vi "Test All Drivers.vi"() -> ()   [LabVIEW 2019, in "instrument.Cryostation.lvclass"]
uses:
  instrument.Cryostation.lvclass
  <vilib>/addons/_JKI Toolkits/Caraya/classes/Test/Test.lvclass
  <vilib>/addons/_JKI Toolkits/Caraya/classes/Assert/Assert.lvclass
  <vilib>/addons/_JKI Toolkits/Caraya/classes/Assert/Assert Not Error.vi
  <vilib>/addons/_JKI Toolkits/Caraya/classes/Assert/Assert Not Equal Value_Variant.vi
panel:
  in  "address":string="130.49.180.32"
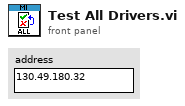
[diagram p1: front panel]
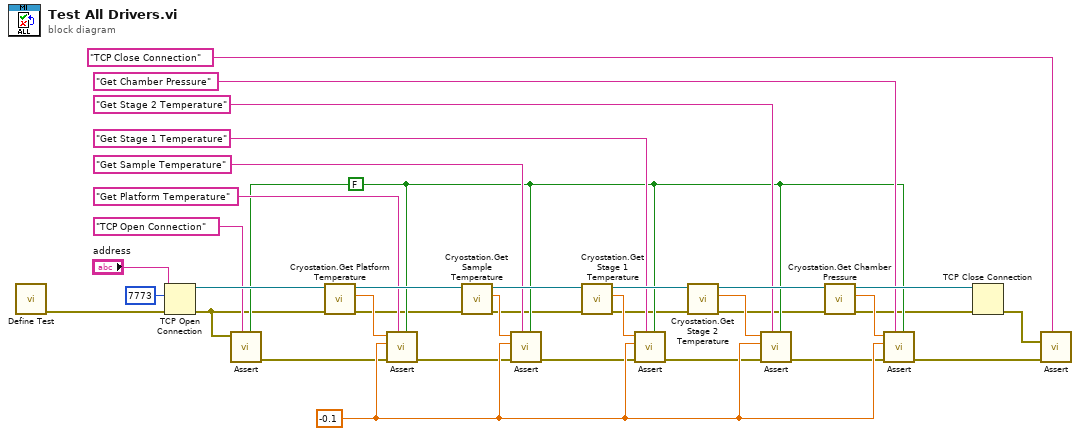
[diagram p0: block diagram]
diagram:
  w16 = FALSE ("Assert Only? (F)")
  w15 = -0.1
  n1 = call <vilib>:"Define Test.vi"() -> ("error out"=w34:errorcluster)  [unwired: 10 in, 1 out]
  n2 = TCP Open Connection(address="address", remote port or service name=u16 7773, error in (no error)=w34) -> (connection ID=w33:refnum<k5>, error out=w4:errorcluster)  [unwired: 2 in]
  n3 = call-poly <vilib>:"Assert.vi"("Assert Only? (F)"=w16, "Label"="TCP Open Connection", "Not Error?"=w4) -> ("error out"=w14:errorcluster)  [unwired: 7 in, 1 out]
  n4 = call "Cryostation.Get Platform Temperature.vi"("error in (no error)"=w4, "TCP Network Connection in"=w33) -> ("error out"=w5:errorcluster, "Platform Temperature (K)"=w17:dbl, "TCP Network Connection out"=w32:refnum<k5>)  [unwired: 7 in]
  n5 = call-poly <vilib>:"Assert.vi"("Assert Only? (F)"=w16, "Label"="Get Platform Temperature", "error in (no error)"=w14, "Actual"=w15, "Expected"=w17) -> ("error out"=w13:errorcluster)  [unwired: 5 in, 1 out]
  n6 = call "Cryostation.Get Sample Temperature.vi"("error in (no error)"=w5, "TCP Network Connection in"=w32) -> ("error out"=w6:errorcluster, "Sample Temperature (K)"=w18:dbl, "TCP Network Connection out"=w31:refnum<k5>)  [unwired: 7 in]
  n7 = call-poly <vilib>:"Assert.vi"("Assert Only? (F)"=w16, "Label"="Get Sample Temperature", "error in (no error)"=w13, "Actual"=w15, "Expected"=w18) -> ("error out"=w12:errorcluster)  [unwired: 5 in, 1 out]
  n8 = call "Cryostation.Get Stage 1 Temperature.vi"("error in (no error)"=w6, "TCP Network Connection in"=w31) -> ("error out"=w7:errorcluster, "Stage 1 Temperature (K)"=w19:dbl, "TCP Network Connection out"=w30:refnum<k5>)  [unwired: 7 in]
  n9 = call-poly <vilib>:"Assert.vi"("Assert Only? (F)"=w16, "Label"="Get Stage 1 Temperature", "error in (no error)"=w12, "Actual"=w15, "Expected"=w19) -> ("error out"=w11:errorcluster)  [unwired: 5 in, 1 out]
  n10 = call "Cryostation.Get Stage 2 Temperature.vi"("error in (no error)"=w7, "TCP Network Connection in"=w30) -> ("error out"=w8:errorcluster, "Stage 2 Temperature (K)"=w20:dbl, "TCP Network Connection out"=w29:refnum<k5>)  [unwired: 7 in]
  n11 = call-poly <vilib>:"Assert.vi"("Assert Only? (F)"=w16, "Label"="Get Stage 2 Temperature", "error in (no error)"=w11, "Actual"=w15, "Expected"=w20) -> ("error out"=w10:errorcluster)  [unwired: 5 in, 1 out]
  n12 = call "Cryostation.Get Chamber Pressure.vi"("error in (no error)"=w8, "TCP Network Connection in"=w29) -> ("error out"=w9:errorcluster, "Chamber Pressure (mTorr)"=w21:dbl, "TCP Network Connection out"=w28:refnum<k5>)  [unwired: 7 in]
  n13 = call-poly <vilib>:"Assert.vi"("Assert Only? (F)"=w16, "Label"="Get Chamber Pressure", "error in (no error)"=w10, "Actual"=w15, "Expected"=w21) -> ("error out"=w2:errorcluster)  [unwired: 5 in, 1 out]
  n14 = TCP Close Connection(connection ID=w28, error in (no error)=w9) -> (error out=w1:errorcluster)  [unwired: 1 in, 1 out]
  n15 = call-poly <vilib>:"Assert.vi"("Label"="TCP Close Connection", "error in (no error)"=w2, "Not Error?"=w1) -> ()  [unwired: 7 in, 2 out]
